vi "Go_to_Shutdown.vi"(8 "error in (no error)":errorcluster, 10 "Cluster in":T2, 11 "Enum in":T1) -> (0 "error out":errorcluster, 1 "Stop State Machine":bool=TRUE, 2 "Cluster out":T2, 3 "Enum out":T1)   [LabVIEW 2018]
uses:
  Type_Def/Type_Def Actuator Controls.ctl
  Type_Def/Type_Def ControlState.ctl
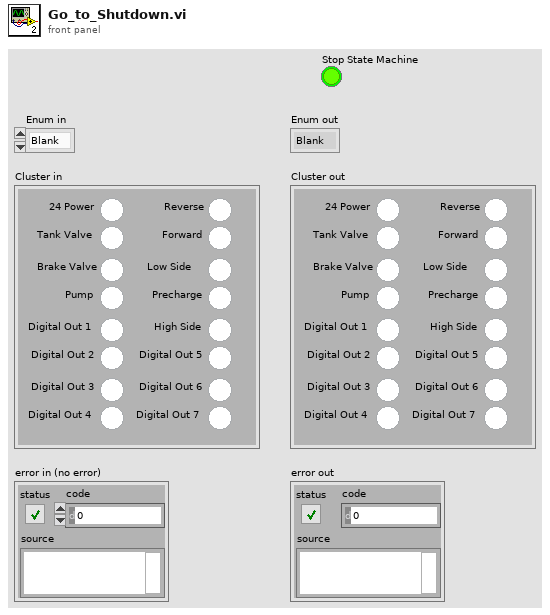
[diagram p1: front panel]
types:
  T1 = typedef "Type_Def ControlState.ctl" = enum16{"Blank", "Systems Check", "Idle", "Ready", "Pushing", "CrawlingPrecharge", "Braking", "Fault", "Boot Up", "Unpowered", "Crawling", "Shutdown", "Service Push", "Service Wait", "Vent", "Precharge", "Cooldown"}
  T2 = typedef "Type_Def Actuator Controls.ctl" = cluster{"Reverse ":bool, "Forward":bool, "Low Side":bool, "Precharge":bool, "High Side":bool, "Digital Out 5":bool, "Digital Out 6":bool, "Digital Out 7 ":bool, "24 Power":bool, "Tank Valve ":bool, "Brake Valve":bool, "Pump":bool, "Digital Out 1 ":bool, "Digital Out 2":bool, "Digital Out 3":bool, "Digital Out 4 ":bool}
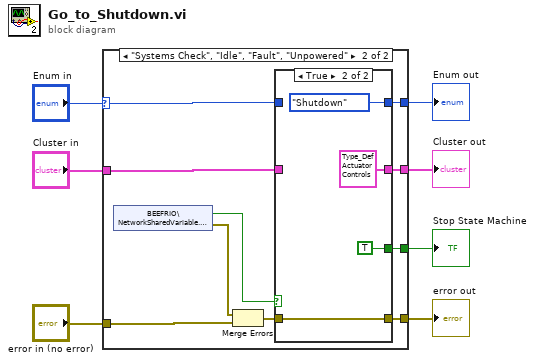
[diagram p0: block diagram]
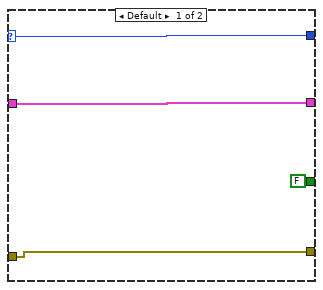
[diagram p2: hidden frame]
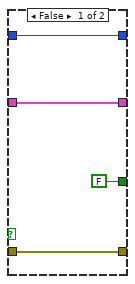
[diagram p3: hidden frame]
diagram:
  n1 = case shown="\"Systems Check\", \"Idle\", \"Fault\", \"Unpowered\"" "Enum in" {
    selector: "Enum in" -> [w11 w17]
    tunnel: "error in (no error)" -> [w9 w14]
    tunnel: "Cluster in" -> [w10 w21]
    tunnel: [w11 w18] -> w5
    tunnel: [w10 w20] -> w4
    tunnel: [w9 w19] -> w3
    tunnel: [FALSE w16] -> w1
    frame Default {
    }
    frame "Systems Check", "Idle", "Fault", "Unpowered" {
      n2 = shared-variable "BEEFRIO\\NetworkSharedVariable.lvlib\\Shutdown"() -> (w15:bool, error out=w13:errorcluster)  [unwired: 1 in]
      n3 = Merge Errors(w13, w14) -> (w12:errorcluster)
      n4 = case shown="True" w15 {
        tunnel: [w25 T2 {"Reverse "=FALSE, "Forward"=FALSE, "Low Side"=FALSE, "Precharge"=FALSE, "High Side"=FALSE, "Digital Out 5"=FALSE, "Digital Out 6"=FALSE, "Digital Out 7 "=FALSE, "24 Power"=FALSE, "Tank Valve "=FALSE, "Brake Valve"=FALSE, "Pump"=FALSE, "Digital Out 1 "=FALSE, "Digital Out 2"=FALSE, "Digital Out 3"=FALSE, "Digital Out 4 "=FALSE} ("Cluster in")] -> w20
        tunnel: w21 -> [w25 _]
        tunnel: [w24 w27] -> w19
        tunnel: w12 -> [w24 w27]
        tunnel: [w23 Type_Def_ControlState."Shutdown" ("Enum in")] -> w18
        tunnel: w17 -> [w23 _]
        tunnel: [FALSE TRUE] -> w16
        frame False {
        }
        frame True {
        }
      }
    }
  }
  "error out" <- w3
  "Cluster out" <- w4
  "Enum out" <- w5
  "Stop State Machine" <- w1
